vi "Convert Fcurve volts.vi"(0 "reference in":refnum<class "XYgraph.lvclass">, 5 "error in (no error)":errorcluster, 9 "X scale Offset":dbl, 11 "Y scale Offset":dbl) -> (14 "reference out":refnum<class "XYgraph.lvclass">, 19 "error out":errorcluster)   [LabVIEW 2019, in "XYgraph.lvclass"]
doc: "Converts the Force curve units using the inverse of the x and y multiplier set in Convert Fcurve units.vi"
uses:
  XYgraph.lvclass
  <vilib>/Utility/miscctls.llb/LVOffsetAndMultiplierTypeDef.ctl
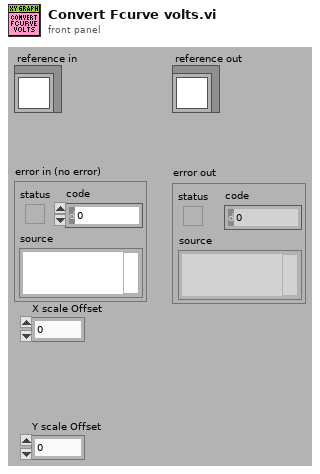
[diagram p1: front panel]
types:
  T1 = typedef "LVOffsetAndMultiplierTypeDef.ctl" = cluster{"Offset":dbl, "Multiplier":dbl}
  T2 = typedef "XYgraph.lvclass/ObjectAttributes.ctl" = cluster{"FPref":T3, "MyAttribute":dbl, "X multiplier":dbl, "Y multiplier":dbl, "X Scale name":string, "Y Scale name":string, "Fcurve metadata":T4, "Fcurve":refnum<class "Fcurve.lvclass">}
  T3 = typedef "XYgraph.lvclass/XY graph ref.ctl" = refnum<vi>
  T4 = typedef "Fcurve.lvclass/Metadata.ctl" = cluster{"dt (us)":dbl, "Dec Factor":dbl, "Z piezo Sensitivity (nm/V)":dbl, "K (N/m)":dbl, "Sp (V)":dbl, "Contact (ms)":dbl, "Zpos contact":dbl, "Vel_app (nm/s)":dbl, "Vel_ret (nm/s)":dbl, "deltaV (nm)":dbl, "Def_V0 (v)":dbl, "Piezo gain":dbl, "invOLS (nm/V)":dbl}
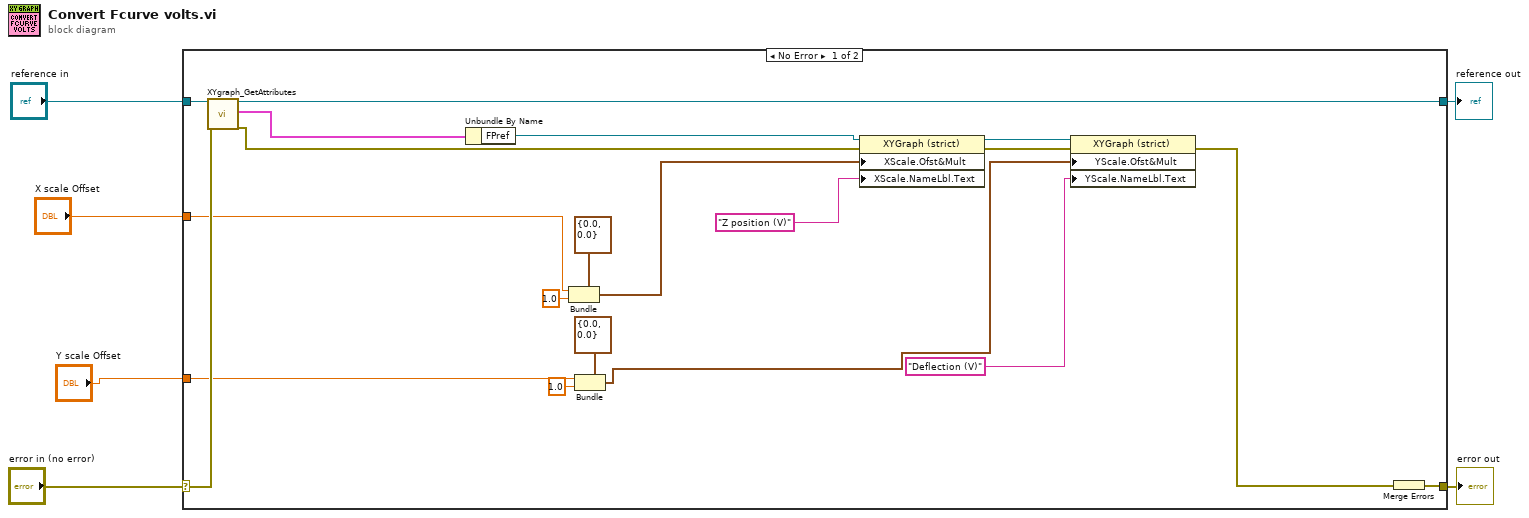
[diagram p0: block diagram]
diagram:
  n1 = case shown="No Error" "error in (no error)" {
    selector: "error in (no error)" -> [w26 w28]
    tunnel: [w19 w28] -> w5
    tunnel: [w10 w27] -> w3
    tunnel: "reference in" -> [w25 w27]
    tunnel: "Y scale Offset" -> [w21 _]
    tunnel: "X scale Offset" -> [w20 _]
    frame No Error {
      n2 = call "XYgraph_GetAttributes.vi"("reference in"=w25, "error in (no error)"=w26) -> ("reference out"=w10:refnum<class "XYgraph.lvclass">, "attributes"=w8:T2, "error out"=w9:errorcluster)  [unwired: 14 in, 1 out]
      n3 = Unbundle By Name(w8) -> ("FPref"=w7:T3)
      n4 = Bundle(cluster=T1 {"Offset"=0.0, "Multiplier"=0.0} ("X Scale.Offset and Multiplier"), "Offset"=w20, "Multiplier"=1.0) -> (w24:T1)
      n5 = Bundle(cluster=T1 {"Offset"=0.0, "Multiplier"=0.0} ("Y Scale.Offset and Multiplier"), "Offset"=w21, "Multiplier"=1.0) -> (w11:T1)
      n6 = property on="Property Node" class="XYGraph (strict)"(reference=w7, error in=w9, "XScale.Ofst&Mult"=w24, "XScale.NameLbl.Text"="Z position (V)" ("X Scale.Name Label.Text")) -> (reference out=w15:T3, error out=w14:errorcluster)
      n7 = property on="Property Node" class="XYGraph (strict)"(reference=w15, error in=w14, "YScale.Ofst&Mult"=w11, "YScale.NameLbl.Text"="Deflection (V)" ("Y Scale.Unit Label.Text")) -> (error out=w13:errorcluster)  [unwired: 1 out]
      n8 = Merge Errors(w13) -> (w19:errorcluster)
    }
    frame Error {
    }
  }
  "error out" <- w5
  "reference out" <- w3
